vi "nodeInfo.get_node_name.vi"(5 "error in (no error)":errorcluster) -> (16 "nodeName":string, 19 "error out":errorcluster)   [LabVIEW 2012, in "LVNodeInfo.lvlib"]
doc: "Gets the name of the node."
uses:
  LVNodeInfo.lvlib
  NodeMon/bin/libNodeInfo.dll
  NodeMon/bin/libNodeInfo.so
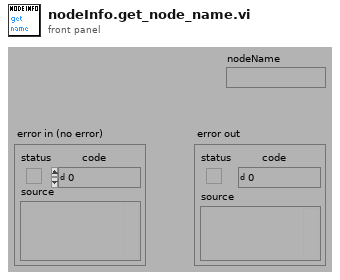
[diagram p1: front panel]
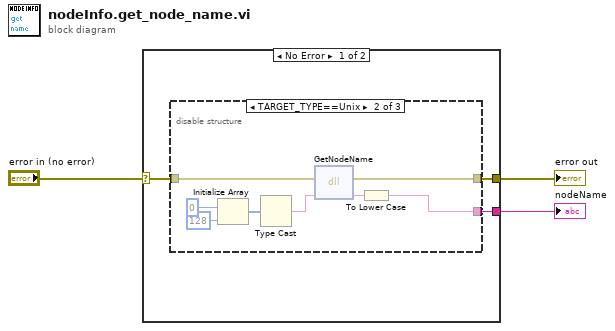
[diagram p0: block diagram]
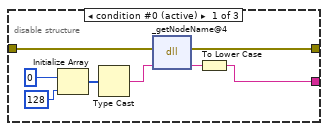
[diagram p2: hidden frame]
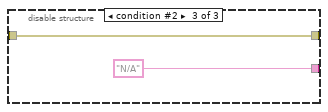
[diagram p3: hidden frame]
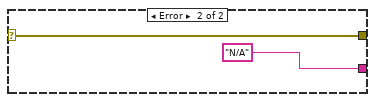
[diagram p4: hidden frame]
diagram:
  n1 = case shown="No Error" "error in (no error)" {
    selector: "error in (no error)" -> [w5 w25]
    tunnel: [w6 "N/A" ("nodeName")] -> w3
    tunnel: [w4 w25] -> w1
    frame No Error {
      n2 = disable-structure "Conditional Disable Structure" shown="TARGET_TYPE==Unix" {
        disable-tunnel: [w9 w17 "N/A"] -> w6
        disable-tunnel: w5 -> [w8 w16 w23]
        disable-tunnel: [w7 w15 w23] -> w4
        frame condition #0 (active) {
          n3 = Initialize Array(i8 0, 128 ("dimension size")) -> (w11:i8[])
          n4 = Type Cast(x=w11) -> (*(type *) &x=w10:string)  [unwired: 1 in]
          n5 = dll-call lib="D:/DIMLVEvent LV2012/NodeMon/bin/libNodeInfo.dll" fn="_getNodeName@4" label="getNodeName"(error in=w8, "nodeName"=w10) -> (error out=w7:errorcluster, "nodeName"=w14:string)  [unwired: 3 in, 1 out]
          n6 = To Lower Case(string=w14) -> (all lower case string=w9:string)
        }
        frame condition #1 {
          n7 = Initialize Array(i8 0, 128 ("dimension size")) -> (w19:i8[])
          n8 = Type Cast(x=w19) -> (*(type *) &x=w18:string)  [unwired: 1 in]
          n9 = dll-call lib="D:/DIMLVEvent LV2012/NodeMon/bin/libNodeInfo.so" fn="GetNodeName"(error in=w16, "nodeName"=w18) -> (error out=w15:errorcluster, "nodeName"=w22:string)  [unwired: 3 in, 1 out]
          n10 = To Lower Case(string=w22) -> (all lower case string=w17:string)
        }
        frame condition #2 {
        }
      }
    }
    frame Error {
    }
  }
  "nodeName" <- w3
  "error out" <- w1
